vi "dvp Vi Get Output Io Function.vi"(9 "pOutputIoFunction":u32(ring) items=["OUTPUT_FUNCTION_NORMAL", "OUTPUT_FUNCTION_STROBE"], 10 "outputIo":u32(ring)=1 items=["OUTPUT_IO_1"=1, "OUTPUT_IO_2"=2, "OUTPUT_IO_3"=3, "OUTPUT_IO_4"=4, "OUTPUT_IO_5"=5, "OUTPUT_IO_6"=6, "OUTPUT_IO_7"=7, "OUTPUT_IO_8"=8], 11 "handle":u32) -> (1 "pOutputIoFunction out":u32(ring) items=["OUTPUT_FUNCTION_NORMAL", "OUTPUT_FUNCTION_STROBE"], 3 "function return":u32(ring))   [LabVIEW 2018, in "LabViewDVPCamera.lvlib"]
doc: "LabviewDvp2Api dvpStatus dvpViGetOutputIoFunction(dvpHandle handle, dvpOutputIo outputIo, dvpOutputIoFunction *pOutputIoFunction);"
uses:
  LabViewDVPCamera.lvlib
  LabViewDVPCamera/LabViewDVPCamera.dll
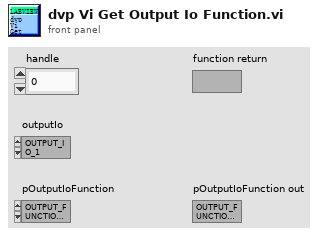
[diagram p1: front panel]
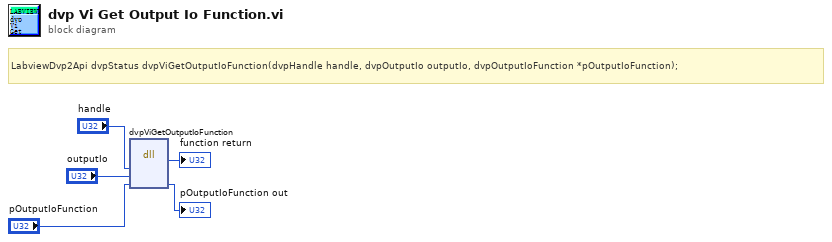
[diagram p0: block diagram]
diagram:
  # "LabviewDvp2Api dvpStatus dvpViGetOutputIoFunction(dvpHandle handle, dvpOutputIo outputIo, dvpOutputIoFunction *pOutputIoFunction);"
  n1 = dll-call lib="C:/Program Files (x86)/DVP2 Labview cn 64/Sample/LabViewDVPCamera/LabViewDVPCamera.*" fn="dvpViGetOutputIoFunction"("handle"="handle", "outputIo"="outputIo", "pOutputIoFunction"="pOutputIoFunction") -> (→"function return":u32, "pOutputIoFunction"=→"pOutputIoFunction out":u32)  [unwired: 5 in, 2 out]
